vi "基于Matlab的音频波形处理与分析 - 3.vi"() -> ()   [LabVIEW 2013]
uses:
  <vilib>/sound2/lvsound2.llb/Sound Data Format.ctl
  <vilib>/sound2/lvsound2.llb/Sampling Mode.ctl
  <vilib>/sound2/lvsound2.llb/Sound File Write Open.vi
  <vilib>/sound2/lvsound2.llb/Sound Input Read (DBL).vi
  <vilib>/sound2/lvsound2.llb/Sound File Write (DBL).vi
  <vilib>/sound2/lvsound2.llb/Sound File Read Open.vi
  <vilib>/sound2/lvsound2.llb/Sound File Read (DBL).vi
  <vilib>/Waveform/WDTOps.llb/WDT Index Channel DBL.vi
panel:
  in  "规定为2D 2":dbl[][](array[numeric])
  in  "退出":bool
  in  "选项卡控件":enum32{"录音系统", "播放系统", "音频处理系统"}(tab)
  in  "停止时间":timestamp format="%<%.1X\n%x>T"
  out "录制时间：":dbl format="%<%H:%M:%S%1u>t"
  in  "设定时间(s)":dbl
  in  "录制方式":enum16{"自由录制", "定时录制", "到点停止"}(ring)
  out "Waveform Graph":waveform(dbl)[](graph) caption="实时波形显示："
  in  "Number of Samples/ch":i32=10000 caption="每通道采样数"
  in  "Device ID":u32 caption="设备 ID" format="%.0x"
  in  "File Path":path=path "test.wav" caption="录音保存在："
  in  "开始按钮":bool
  in  "停止":bool
  in  "sound format":T1={"sample rate (S/s)"=22050.0, "number of channels"=2, "bits per sample"=16} caption="声音格式"
  in  "停止播放":bool
  in  "打开要播放的WAV文件":path=path "C:/WINDOWS/Media/TADA.WAV" caption="sound"
  in  "设备 ID":u32 caption="Device ID" format="%.0x"
  out "Waveform Graph 2":waveform(dbl)[](graph) caption="实时波形显示："
  in  "播放按钮":bool
  out "播放时间：":dbl format="%<%H:%M:%S%1u>t"
  in  "规定为2D":dbl[][](array[numeric])
  in  "查询":dbl
  out "查询音频":dbl[](graph)
  in  "要处理的音频：":path
  in  "确定按钮":bool
  out "数据文件":refnum<file>
  out "总体类型估计":dbl[](graph)
  out "查询类型":dbl[](graph)
  in  "停止检索":bool
  out "人声时间":dbl
  out "数传音时间":dbl
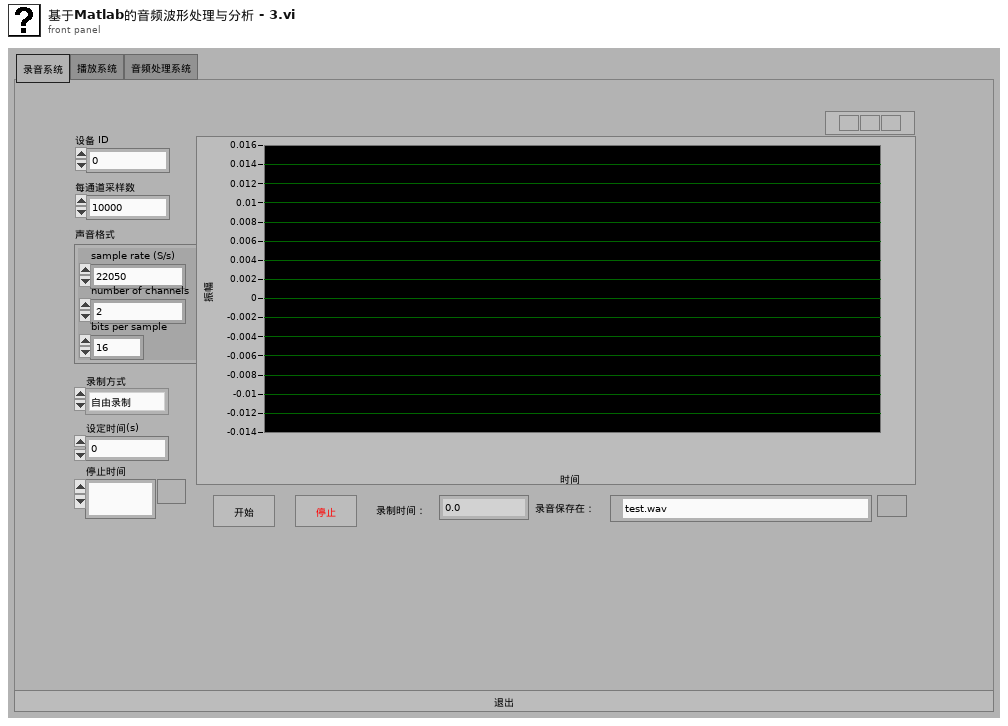
[diagram p1: front panel]
types:
  T1 = typedef "Sound Data Format.ctl" = cluster{"sample rate (S/s)":dbl, "number of channels":i32, "bits per sample":i32}
  T2 = typedef "Sound File Refnum.ctl" = refnum<file>
  T3 = typedef "Sampling Mode.ctl" = i32
  T4 = typedef "Sound Input Task ID.ctl" = u32
  T5 = typedef "Sound Output Task ID.ctl" = u32
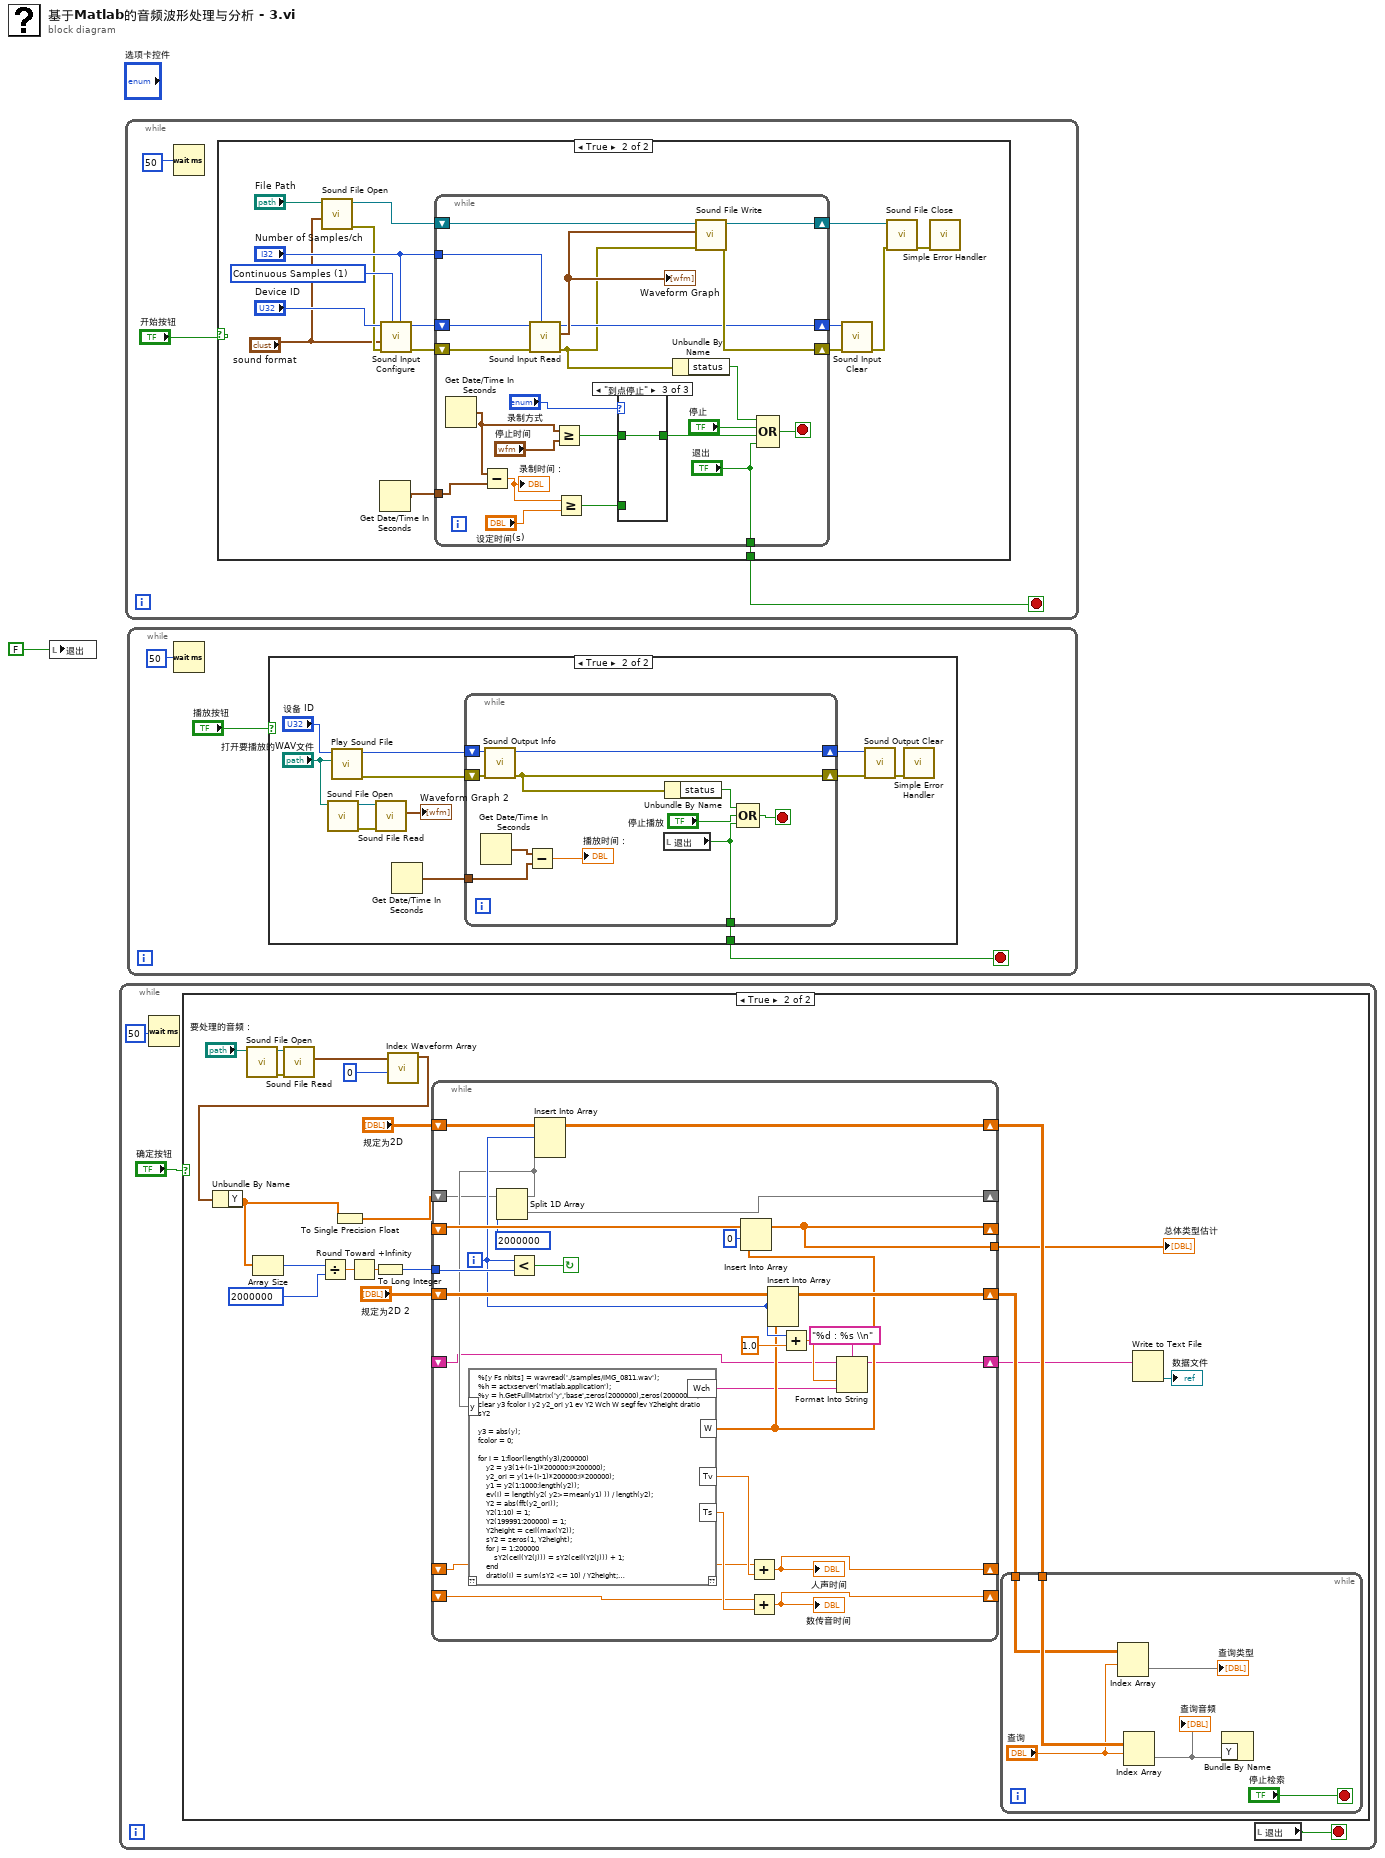
[diagram p0: block diagram]
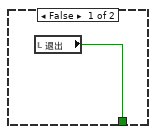
[diagram p3: hidden frame]
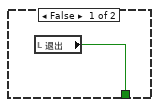
[diagram p4: hidden frame]
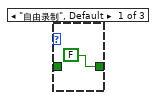
[diagram p5: hidden frame]
diagram:
  n1 = local write "退出"(FALSE) -> ()
  n2 = while {
    stop <- w3 stop-if-true
    n3 = Wait (ms)(milliseconds to wait=50) -> ()  [unwired: 1 out]
    n4 = case shown="True" "确定按钮" {
      frame False {
      }
      frame True {
        n5 = call-poly <vilib>:"Sound File Open.vi"("path"="要处理的音频：") -> ("error out"=w20:errorcluster, "sound file refnum"=w23:T2)  [unwired: 9 in]
        n6 = call-poly <vilib>:"Sound File Read.vi"("error in (no error)"=w20, "sound file refnum"=w23) -> ("data"=w21:waveform(dbl)[])  [unwired: 5 in, 4 out]
        n7 = call-poly <vilib>:"Index Waveform Array.vi"("index"=0, "waveform array"=w21) -> ("waveform"=w17:waveform(dbl))  [unwired: 8 in, 1 out]
        n8 = Unbundle By Name(w17) -> ("Y"=w8:dbl[])
        n9 = Array Size(array=w8) -> (size(s)=w16:i32)
        n10 = Divide(x=w16, y=2000000) -> (x/y=w14:dbl)
        n11 = To Single Precision Float(number=w8) -> (single precision float=w7:sgl[])
        n12 = Round Toward +Infinity(x=w14) -> (ceil(x): smallest int >= x=w13:dbl)
        n13 = To Long Integer(number=w13) -> (32bit integer=w12:i32)
        n14 = while {
          shift-right: [w43] -> _
          shift-left: w7 -> [w42]
          tunnel: w12 -> [w56]
          shift-right: [w52] -> _
          shift-left: _ -> [w53]
          tunnel: [w52] -> w9
          shift-right: [w51] -> w18
          shift-left: "规定为2D 2" -> [w50]
          shift-right: [w55] -> w19
          shift-left: "规定为2D" -> [w41]
          shift-right: [w38] -> _
          shift-left: _ -> [w37]
          shift-right: [w36] -> _
          shift-left: _ -> [w35]
          shift-right: [w32] -> w5
          shift-left: _ -> [w31]
          i -> [w48]
          stop <- w57 continue-if-true
          n15 = Split 1D Array(array=w42, index=2000000) -> (first subarray=w46:sgl[], second subarray=w43:sgl[])
          n16 = script code="%[y Fs nbits] = wavread('./samples/IMG_0811.wav');\n%h = actxserver('matlab.application');\n%y = h.GetFullMatrix('y','base',zeros(2000000),zeros(2000000));\nclear y3 fcolor i y2 y2_ori y1 ev Y2 Wch W segf fev Y2height dratio sY2\n\ny3 = abs(y);\nfcolor = 0;\n\nfor i = 1:floor(length(y3)/200000)\n    y2 = y3(1+(i-1)*200000:i*200000);\n    y2_ori = y(1+(i-1)*200000:i*200000);\n    y1 = y2(1:1000:length(y2));\n    ev(i) = length(y2( y2>=mean(y1) )) / length(y2);\n    Y2 = abs(fft(y2_ori));\n    Y2(1:10) = 1;\n    Y2(199991:200000) = 1;\n    Y2height = ceil(max(Y2));\n    sY2 = zeros(1, Y2height);\n    for j = 1:200000\n        sY2(ceil(Y2(j))) = sY2(ceil(Y2(j))) + 1;\n    end\n    dratio(i) = sum(sY2 <= 10) / Y2height;\n    if ev(i) < 0.375\n        if dratio(i) < 0.88\n            Wch(i) = 'v';\n            W(i) = 0;\n        else\n            Wch(i) = 's';\n            W(i) = 1;\n        end\n    else\n        if dratio(i) <= 0.5\n            Wch(i) = 'n';\n            W(i) = 2;\n        else\n            segf = Y2(6000:100000-1);\n            if (length(segf( segf < 10 )) / length(segf)) >= 0.95\n            Wch(i) = 'n';\n            W(i) = 2;\n            else\n            Wch(i) = 's';\n            W(i) = 1;\n            end\n        end\n    end\nend\n\nTv = sum( W==0 )*200000/44100;\nTs = sum( W==1 )*200000/44100;\n\ny1 = y3(1:1000:length(y3));\nfev = length(y3( y3>=mean(y1) )) / length(y3);\nif fev >= 0.375\n    fcolor = 1;\nend\n\n%h.PutWorkspaceData('W', 'base', W);\n%h.PutWorkspaceData('Tv', 'base', Tv);\n%h.PutWorkspaceData('Ts', 'base', Ts);\n%h.PutWorkspaceData('fcolor', 'base', fcolor);\n%h.PutCharArray('Wch', 'base', Wch);"("y"=w46) -> ("W"=w45:dbl[], "Wch"=w33:string, "Tv"=w39:dbl, "Ts"=w40:dbl)  [unwired: 1 in, 1 out]
          n17 = Less?(x=w48, y=w56) -> (x < y?=w57:bool)
          n18 = Insert Into Array(array=w41, index (row)=w48, new element=w46) -> (w55:dbl[][])  [unwired: 1 in]
          n19 = Insert Into Array "Insert Into Array"(array=w53, index=0, new element=w45) -> (w52:dbl[])
          n20 = Add(x=w37, y=w39) -> (x+y=w38:dbl)
          "人声时间" <- w38
          n21 = Add(x=w35, y=w40) -> (x+y=w36:dbl)
          "数传音时间" <- w36
          n22 = Insert Into Array(array=w50, index (row)=w48, new element=w45) -> (w51:dbl[][])  [unwired: 1 in]
          n23 = Add(x=w48, y=1.0) -> (x+y=w47:dbl)
          n24 = Format Into String(format string="%d : %s \\n", initial string=w31, w47, w33) -> (resulting string=w32:string)  [unwired: 1 in, 1 out]
        }
        "总体类型估计" <- w9
        n25 = while {
          tunnel: w19 -> [w30]
          tunnel: w18 -> [w29]
          stop <- "停止检索" stop-if-true
          n26 = Index Array(array=w29, index (row)="查询") -> (element=→"查询类型":dbl[])  [unwired: 1 in]
          n27 = Index Array(array=w30, index (row)="查询") -> (element=w25:dbl[])  [unwired: 1 in]
          "查询音频" <- w25
          n28 = Bundle By Name("Y"=w25) -> ()  [unwired: 1 in, 1 out]
        }
        n29 = Write to Text File(text=w5) -> (refnum out=→"数据文件":refnum<file>)  [unwired: 3 in, 2 out]
      }
    }
    n30 = local read "退出"() -> (w3:bool)
  }
  n31 = while {
    stop <- w58 stop-if-true
    n32 = Wait (ms)(milliseconds to wait=50) -> ()  [unwired: 1 out]
    n33 = case shown="True" "开始按钮" {
      tunnel: [w61 w64] -> w58
      frame False {
        n34 = local read "退出"() -> (w61:bool)
      }
      frame True {
        w70 = T3 1 items=["Finite Samples", "Continuous Samples"] ("sample mode")
        n35 = call-poly <vilib>:"Sound File Open.vi"("sound format"="sound format", "path"="File Path") -> ("error out"=w66:errorcluster, "sound file refnum"=w69:T2)  [unwired: 8 in]
        n36 = Get Date/Time In Seconds() -> (seconds since 1Jan1904=w62:timestamp)
        n37 = call <vilib>:"Sound Input Configure.vi"("number of samples/ch"="Number of Samples/ch", "sample mode"=w70, "error in (no error)"=w66, "sound format"="sound format", "device ID"="Device ID") -> ("error out"=w77:errorcluster, "task ID"=w75:T4)  [unwired: 5 in]
        n38 = while {
          tunnel: "Number of Samples/ch" -> [w97]
          shift-right: [w95] -> w68
          shift-left: w69 -> [w96]
          shift-right: [w92] -> w74
          shift-left: w75 -> [w98]
          shift-right: [w94] -> w73
          shift-left: w77 -> [w99]
          tunnel: ["退出"] -> w64
          tunnel: w62 -> [w88]
          stop <- w78 stop-if-true
          n39 = Get Date/Time In Seconds() -> (seconds since 1Jan1904=w85:timestamp)
          n40 = Subtract(x=w85, y=w88) -> (x-y=w86:dbl)
          "录制时间：" <- w86
          n41 = call-poly <vilib>:"Sound Input Read.vi"("number of samples/ch"=w97, "error in (no error)"=w99, "task ID"=w98) -> ("error out"=w91:errorcluster, "data"=w93:waveform(dbl)[], "task ID out"=w92:T4)  [unwired: 6 in]
          "Waveform Graph" <- w93
          n42 = Greater Or Equal?(x=w85, y="停止时间") -> (x >= y?=w81:bool)
          n43 = Greater Or Equal?(x=w86, y="设定时间(s)") -> (x >= y?=w82:bool)
          n44 = case shown="\"到点停止\"" "录制方式" {
            tunnel: w82 -> [_ w101 _]
            tunnel: w81 -> [_ _ w102]
            tunnel: [FALSE w101 w102] -> w79
            frame "自由录制", Default {
            }
            frame "定时录制" {
            }
            frame "到点停止" {
            }
          }
          n45 = Unbundle By Name(w91) -> ("status"=w90:bool)
          n46 = call-poly <vilib>:"Sound File Write.vi"("error in (no error)"=w91, "data"=w93, "sound file refnum"=w96) -> ("error out"=w94:errorcluster, "sound file refnum out"=w95:T2)  [unwired: 7 in]
          n47 = Compound Arithmetic op=OR(w90, "停止", w79, "退出") -> (w78:bool)
        }
        n48 = call <vilib>:"Sound Input Clear.vi"("error in (no error)"=w73, "task ID"=w74) -> ("error out"=w67:errorcluster)  [unwired: 9 in]
        n49 = call <vilib>:"Sound File Close.vi"("error in (no error)"=w67, "sound file refnum"=w68) -> ("error out"=w65:errorcluster)  [unwired: 9 in]
        n50 = call <vilib>:"Simple Error Handler.vi"("error in (no error)"=w65) -> ()  [unwired: 4 in, 5 out]
      }
    }
  }
  n51 = while {
    stop <- w103 stop-if-true
    n52 = Wait (ms)(milliseconds to wait=50) -> ()  [unwired: 1 out]
    n53 = case shown="True" "播放按钮" {
      tunnel: [w106 w107] -> w103
      frame False {
        n54 = local read "退出"() -> (w106:bool)
      }
      frame True {
        n55 = call-poly <vilib>:"Sound File Open.vi"("path"="打开要播放的WAV文件") -> ("error out"=w113:errorcluster, "sound file refnum"=w112:T2)  [unwired: 9 in]
        n56 = call <vilib>:"Play Sound File.vi"("path"="打开要播放的WAV文件", "device ID"="设备 ID") -> ("error out"=w109:errorcluster, "task ID"=w110:T5)  [unwired: 8 in]
        n57 = call-poly <vilib>:"Sound File Read.vi"("error in (no error)"=w113, "sound file refnum"=w112) -> ("data"=→"Waveform Graph 2":waveform(dbl)[])  [unwired: 5 in, 4 out]
        n58 = Get Date/Time In Seconds() -> (seconds since 1Jan1904=w108:timestamp)
        n59 = while {
          shift-right: [w128] -> w115
          shift-left: w109 -> [w126]
          shift-right: [w129] -> w116
          shift-left: w110 -> [w127]
          tunnel: w108 -> [w124]
          tunnel: [w119] -> w107
          stop <- w122 stop-if-true
          n60 = Get Date/Time In Seconds() -> (seconds since 1Jan1904=w125:timestamp)
          n61 = call <vilib>:"Sound Output Info.vi"("error in (no error)"=w126, "task ID"=w127) -> ("error out"=w128:errorcluster, "task ID out"=w129:T5)  [unwired: 6 in, 2 out]
          n62 = Subtract(x=w125, y=w124) -> (x-y=→"播放时间：":dbl)
          n63 = local read "退出"() -> (w119:bool)
          n64 = Unbundle By Name(w128) -> ("status"=w121:bool)
          n65 = Compound Arithmetic op=OR(w121, "停止播放", w119) -> (w122:bool)
        }
        n66 = call <vilib>:"Sound Output Clear.vi"("error in (no error)"=w115, "task ID"=w116) -> ("error out"=w118:errorcluster)  [unwired: 9 in]
        n67 = call <vilib>:"Simple Error Handler.vi"("error in (no error)"=w118) -> ()  [unwired: 4 in, 5 out]
      }
    }
  }
